vi "SwerveMath.vi"() -> ()   [LabVIEW 2015]
uses:
  2015RobotCode/Robot Global Data.vi
panel:
  in  "Rotation Angle Cluster":dbl
  in  "Rotation Multipliers":dbl
  out "Motor Angles":dbl[](array[numeric])
  out "Motor Speeds":dbl[](array[numeric])
  in  "Angle (degrees; 0 = right)":dbl
  in  "FieldCentric? (T)":bool=TRUE
  in  "Strafe Joystick Axes":cluster{"X":dbl, "Y":dbl}
  in  "Trigger Axes/Turn Speed":cluster{"Left":dbl, "Right":dbl}
  in  "Strafe Multiplier":dbl
  in  "Rotation Multiplier":dbl
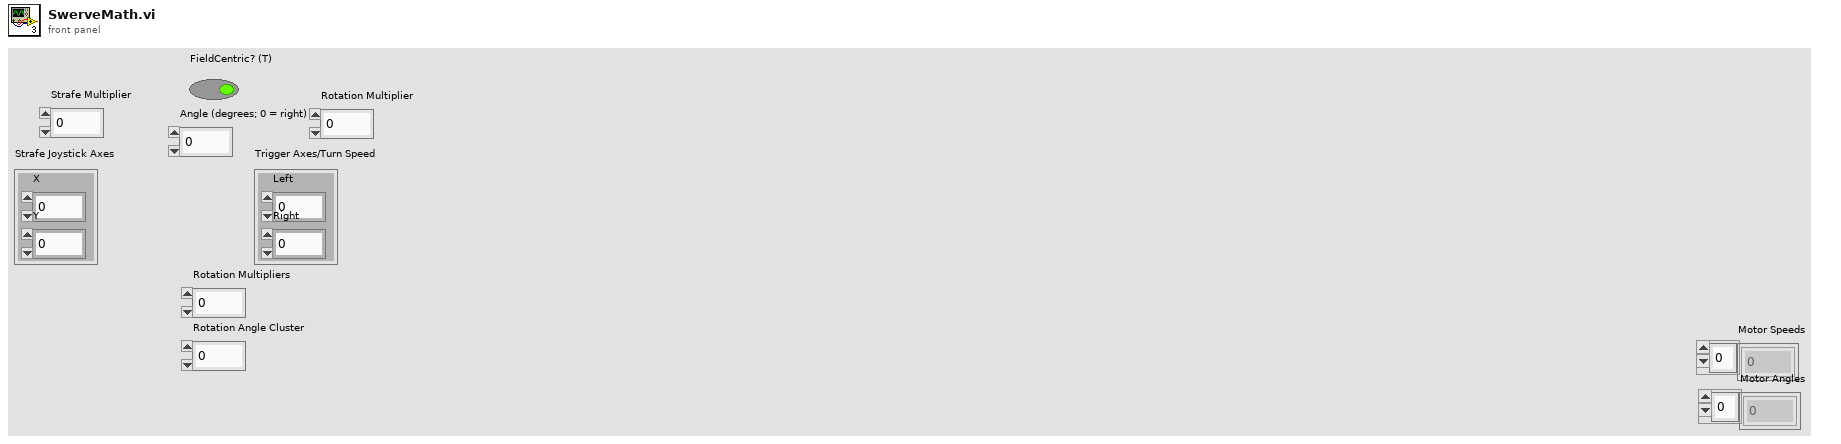
[diagram p1: front panel]
types:
  T1 = cluster{"FL Angle":dbl, "FR Angle":dbl, "RL Angle":dbl, "RR Angle":dbl}
  T2 = cluster{"normalized array[0]":dbl, "normalized array[1]":dbl, "normalized array[2]":dbl, "normalized array[3]":dbl}
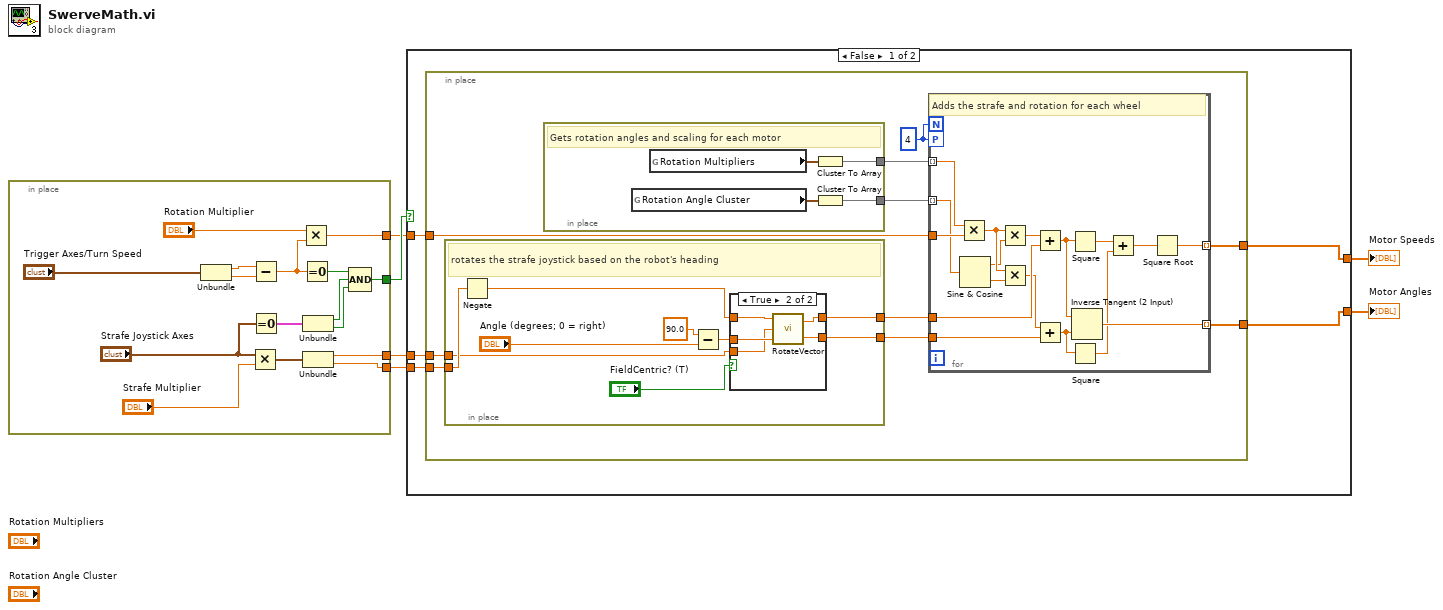
[diagram p0: block diagram]
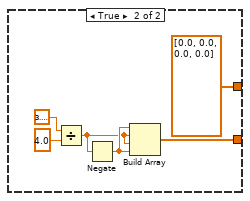
[diagram p3: hidden frame]
diagram:
  n1 = in-place {
    in-place-border: [w15] -> w6
    in-place-border: [w14] -> w5
    in-place-border: [w13] -> w4
    in-place-border: [w11] -> w3
    n2 = Unbundle("Trigger Axes/Turn Speed") -> ("Left"=w18:dbl, "Right"=w19:dbl)
    n3 = Multiply(x="Strafe Joystick Axes", y="Strafe Multiplier") -> (x*y=w9:cluster{"X":dbl, "Y":dbl})
    n4 = Subtract(x=w18, y=w19) -> (x-y=w12:dbl)
    n5 = Equal To 0?(x="Strafe Joystick Axes") -> (x = 0?=w21:cluster{"X":bool, "Y":bool})
    n6 = Multiply(x="Rotation Multiplier", y=w12) -> (x*y=w11:dbl)
    n7 = Equal To 0?(x=w12) -> (x = 0?=w7:bool)
    n8 = Unbundle(w21) -> ("X"=w17:bool, "Y"=w16:bool)
    n9 = Unbundle(w9) -> ("X"=w13:dbl, "Y"=w14:dbl)
    n10 = Compound Arithmetic op=AND(w7, w17, w16) -> (w15:bool)
  }
  n11 = case shown="False" w6 {
    tunnel: w5 -> [w27 _]
    tunnel: w4 -> [w26 _]
    tunnel: w3 -> [w25 _]
    tunnel: [w23 dbl[] [0.0, 0.0, 0.0, 0.0] ("appended array")] -> w2
    tunnel: [w24 w75] -> w1
    frame False {
      n12 = in-place {
        in-place-border: [w35] -> w23
        in-place-border: [w34] -> w24
        in-place-border: w27 -> [w32]
        in-place-border: w26 -> [w31]
        in-place-border: w25 -> [w30]
        w33 = 4
        n13 = in-place {
          in-place-border: [w50] -> w37
          in-place-border: [w49] -> w36
          in-place-border: w32 -> [w45]
          in-place-border: w31 -> [w44]
          # "rotates the strafe joystick based on the robot's heading"
          n14 = Negate(x=w45) -> (-x=w46:dbl)
          n15 = Subtract(x=90.0 ("y"), y="Angle (degrees; 0 = right)") -> (x-y=w47:dbl)
          n16 = case shown="True" "FieldCentric? (T)" {
            tunnel: w46 -> [w52 w57]
            tunnel: [w52 w54] -> w50
            tunnel: [w51 w53] -> w49
            tunnel: w47 -> [_ w56]
            tunnel: w44 -> [w51 w55]
            frame False {
            }
            frame True {
              n17 = call "RotateVector.vi"("Angle"=w56, "X"=w55, "Y"=w57) -> ("X'"=w53:dbl, "Y'"=w54:dbl)
            }
          }
        }
        n18 = in-place {
          in-place-border: [w40] -> w29
          in-place-border: [w41] -> w28
          # "Gets rotation angles and scaling for each motor"
          n19 = global read "Robot Global Data.vi" "Rotation Angle Cluster"() -> (w39:T1)
          n20 = global read "Robot Global Data.vi" "Rotation Multipliers"() -> (w38:T2)
          n21 = Cluster To Array(cluster=w38) -> (array=w40:dbl[])
          n22 = Cluster To Array(cluster=w39) -> (array=w41:dbl[])
        }
        n23 = for {
          N: w33 -> [_]
          tunnel: w37 -> [w74]
          tunnel: w36 -> [w73]
          tunnel: w30 -> [w72]
          tunnel: [w71] -> w35 mode=indexing
          tunnel: [w70] -> w34 mode=indexing
          workers-P: w33 -> [_]
          tunnel: w29 -> [w59] mode=indexing
          tunnel: w28 -> [w58] mode=indexing
          # "Adds the strafe and rotation for each wheel"
          n24 = Multiply(x=w59, y=w72) -> (x*y=w62:dbl)
          n25 = Sine & Cosine(0:w58) -> (1:w61:dbl, 2:w60:dbl)
          n26 = Multiply(x=w62, y=w61) -> (x*y=w65:dbl)
          n27 = Multiply(x=w62, y=w60) -> (x*y=w66:dbl)
          n28 = Add(x=w65, y=w74) -> (x+y=w64:dbl)
          n29 = Add(x=w66, y=w73) -> (x+y=w63:dbl)
          n30 = Square(x=w64) -> (x^2=w68:dbl)
          n31 = Square(x=w63) -> (x^2=w67:dbl)
          n32 = Inverse Tangent (2 Input)(1:w63, 2:w64) -> (0:w70:dbl)
          n33 = Add(x=w68, y=w67) -> (x+y=w69:dbl)
          n34 = Square Root(x=w69) -> (sqrt(x)=w71:dbl)
        }
      }
    }
    frame True {
      n35 = Divide(x=3.141592653589793, y=4.0) -> (x/y=w79:dbl)
      n36 = Negate(x=w79) -> (-x=w80:dbl)
      n37 = Build Array(w80, w79, w79, w80) -> (w75:dbl[])
    }
  }
  "Motor Speeds" <- w2
  "Motor Angles" <- w1
